vi "Panther Dashboard.vi"(8 "error in":errorcluster, 11 "Include Dependencies (T)":bool=TRUE) -> (0 "error out":errorcluster)   [LabVIEW 2020]
uses:
  Panther Dashboard/Panther Dashboard.lvlib
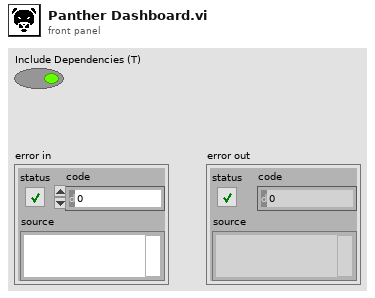
[diagram p1: front panel]
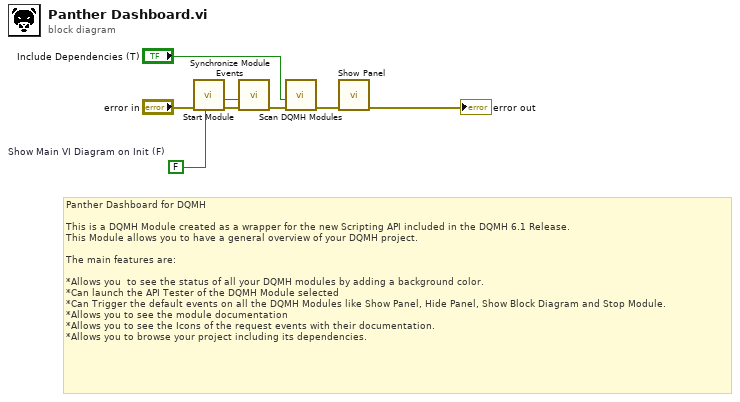
[diagram p0: block diagram]
diagram:
  w1 = FALSE  # Show Main VI Diagram on Init (F)
  # "Panther Dashboard for DQMH\n\nThis is a DQMH Module created as a wrapper for the new Scripting API included in the DQMH 6.1 Release.\nThis Module allows you to have a general overview of your DQMH project.\n\nThe main features are:\n\n*Allows you  to see the status of all your DQMH modules by adding a background color.\n*Can launch the API Tester of the DQMH Module selected\n*Can Trigger the default events on all the DQMH Modules like Show Panel, Hide Panel, Show Block Diagram and Stop Module.\n*Allows you to see the module documentation\n*Allows you to see the Icons of the request events with their documentation.\n*Allows you to browse your project including its dependencies."
  n1 = call "Start Module.vi"("Show Main VI Diagram on Init (F)"=w1, "error in"="error in") -> ("error out"=w8:errorcluster, "Wait for Event Sync?"=w3:bool)  [unwired: 6 in, 2 out]
  n2 = call "Synchronize Module Events.vi"("error in"=w8, "Wait for Event Sync?"=w3) -> ("error out"=w7:errorcluster)  [unwired: 9 in]
  n3 = call "Scan DQMH Modules.vi"("error in"=w7, "Include Dependencies"="Include Dependencies (T)") -> ("error out"=w6:errorcluster)  [unwired: 9 in]
  n4 = call "Show Panel.vi"("error in (no error)"=w6) -> ("error out"=→"error out":errorcluster)  [unwired: 10 in]
